vi "IMAQDevice.snap.vi"(0 "i ref in":refnum<vi>, 5 "error in (no error)":errorcluster) -> (14 "i ref out":refnum<vi>, 19 "error out":errorcluster)   [LabVIEW 2014, in "IMAQDevice.lvlib"]
doc: "This VI is use in the one-shot mode to capture a picture, which will be saved in the image attribute of the CS class.\n\nLicense Agreement for this software:\n\nCopyright (C)\nGesellschaft für Schwerionenforschung, GSI\nPlanckstr. 1\n64291 Darmstadt\nGermany\n\nContact: D.Beck@gsi.de \n\nThis program is free software; you can redistribute it and/or modify it under the terms of the \nGNU General Public License as published by the Free Software Foundation; either version 2 of \nthe license, or (at your option) any later version.\n\nThis program is distributed in the hope that it will be useful, but WITHOUT ANY WARRANTY; \nwithout even the implied warranty of MERCHANTABILITY or FITNESS FOR A PARTICULAR PURPOSE. See the GNU General License for more details (http://www.gnu.org).\n\nGesellschaft für Schwerionenforschung, GSI\nPlanckstr. 1, 64291 Darmstadt, Germany\nFor all questions and ideas contact: M.Richter@gsi.de, H.Brand@gsi.de or D.Beck@gsi.de.\nLast update: 16-JUN-2004"
uses:
  IMAQDevice.lvlib
  CSlibraries-extern/HGF/HGF_LVC/HGF_IMAQ/HGF_IMAQDevice/HGF_IMAQDevice.lvclass
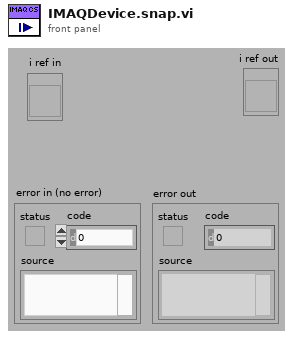
[diagram p1: front panel]
types:
  T1 = typedef "IMAQDevice.lvlib/IMAQDevice.i attribute.ctl" = cluster{"HGF_IMAQ.lvlib:HGF_IMAQDevice.lvclass":refnum<class "HGF_IMAQDevice.lvclass">, "Image":T2, "TimeStampID":i32, "Image IDs":i32[], "NumberOfImagesID":i32, "JPEG?":bool, "JPEGID":i32, "JPEG_ImageID":i32, "TriggerModeID":i32, "OffsetFromLeft":i32, "OffsetFromTop":i32, "HorizontalPixelPerMm":dbl, "VerticalPixelPerMm":dbl, "Grid":cluster{"1":cluster{i32, i32}, "2":cluster{i32, i32}, "3":cluster{i32, i32}, "4":cluster{i32, i32}}, "GridR":cluster{"1":cluster{dbl, dbl}, "2":cluster{dbl, dbl}, "3":cluster{dbl, dbl}, "4":cluster{dbl, dbl}}, "CameraTypeID":i32, "CameraInfos":cluster{"Camera Name-Array":string[], "own Camera Type":string}, "TakeMeasurement?":bool, "TriggerArmedID":i32, "Mirroring":i16, "Rotation":dbl}
  T2 = typedef "IMAQ Image.ctl" = refnum<image>
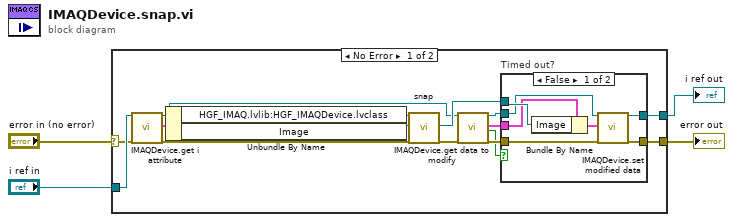
[diagram p0: block diagram]
diagram:
  n1 = case shown="No Error" "error in (no error)" {
    selector: "error in (no error)" -> [w18 w30]
    tunnel: "i ref in" -> [w19 w29]
    tunnel: [w16 w30] -> w2
    tunnel: [w17 w29] -> w1
    frame No Error {
      n2 = call "IMAQDevice.get i attribute.vi"("i ref in"=w19, "error in (no error)"=w18) -> ("i ref out"=w11:refnum<vi>, "i attribute"=w7:T1, "error out"=w13:errorcluster)  [unwired: 15 in]
      n3 = Unbundle By Name(w7) -> ("HGF_IMAQ.lvlib:HGF_IMAQDevice.lvclass"=w12:refnum<class "HGF_IMAQDevice.lvclass">, "Image"=w15:T2)
      n4 = call "snap.vi"("HGF_IMAQDevice"=w12, "Image In"=w15, "error in (no error)"=w13) -> ("Image Out"=w14:T2, "error out"=w8:errorcluster)  [unwired: 14 in, 1 out]
      n5 = call "IMAQDevice.get data to modify.vi"("i ref in"=w11, "error in (no error)"=w8) -> ("i ref out"=w10:refnum<vi>, "i attribute"=w6:T1, "timed out"=w5:bool, "error out"=w9:errorcluster)  [unwired: 14 in]
      n6 = case "Timed out?" shown="False" w5 {
        tunnel: [w26 w28] -> w17
        tunnel: [w25 w27] -> w16
        tunnel: w14 -> [w23 _]
        tunnel: w10 -> [w22 w28]
        tunnel: w9 -> [w21 w27]
        tunnel: w6 -> [w20 _]
        frame False {
          n7 = Bundle By Name(cluster=w20, "Image"=w23) -> (w24:T1)
          n8 = call "IMAQDevice.set modified data.vi"("i ref in"=w22, "i attribute"=w24, "error in (no error)"=w21) -> ("i ref out"=w26:refnum<vi>, "error out"=w25:errorcluster)  [unwired: 15 in]
        }
        frame True {
        }
      }
    }
    frame Error {
    }
  }
  "i ref out" <- w1
  "error out" <- w2
